vi "Set DOF Settings.vi"(6 "Backend engine":T1, 8 "error in":errorcluster, 11 "Degrees Of Freedom":T2={"Required"=TRUE, "Generate"=TRUE}) -> (0 "error out":errorcluster)   [LabVIEW 2013]
doc: "Set calculation settings for Degrees of Freedom."
uses:
  TD DOF Calculation Settings.ctl
  TD Backend Engine.ctl
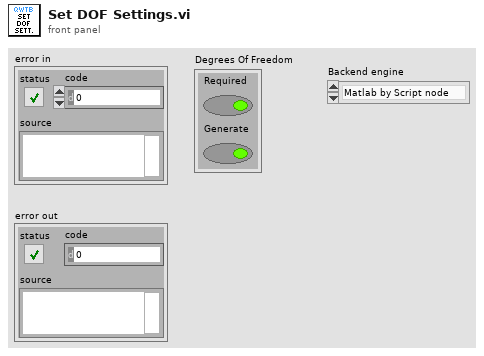
[diagram p1: front panel]
types:
  T1 = typedef "TD Backend Engine.ctl" = enum16{"Matlab by Script node", "GNU Octave by GOLPI"}
  T2 = typedef "TD DOF Calculation Settings.ctl" = cluster{"Required":bool, "Generate":bool}
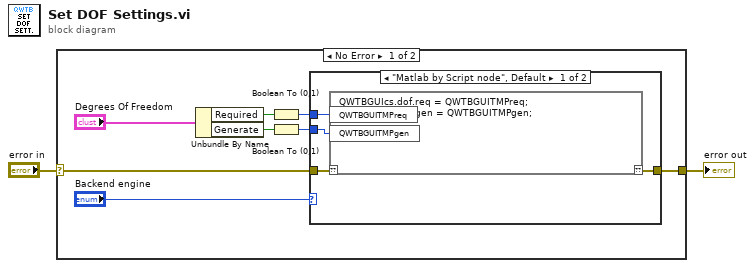
[diagram p0: block diagram]
diagram:
  n1 = case shown="No Error" "error in" {
    selector: "error in" -> [w8 w16]
    tunnel: [w10 w16] -> w2
    frame No Error {
      n2 = Unbundle By Name("Degrees Of Freedom") -> ("Required"=w7:bool, "Generate"=w6:bool)
      n3 = Boolean To (0,1)(Boolean=w7) -> (0, 1=w9:i16)
      n4 = Boolean To (0,1)(Boolean=w6) -> (0, 1=w5:i16)
      n5 = case shown="\"Matlab by Script node\", Default" "Backend engine" {
        tunnel: [w14 w15] -> w10
        tunnel: w9 -> [w13 _]
        tunnel: w5 -> [w11 _]
        tunnel: w8 -> [w12 w15]
        frame "Matlab by Script node", Default {
          n6 = script code="QWTBGUIcs.dof.req = QWTBGUITMPreq;\nQWTBGUIcs.dof.gen = QWTBGUITMPgen;"("??"=w12, "QWTBGUITMPreq"=w13, "QWTBGUITMPgen"=w11) -> ("??"=w14:errorcluster)
        }
        frame "GNU Octave by GOLPI" {
          # "#2DO"
        }
      }
    }
    frame Error {
    }
  }
  "error out" <- w2
